vi "Client Loop Async.vi"(11 "VISA Client in":refnum<class "Serial Client.lvclass">) -> ()   [LabVIEW 2020, in "Stream-Serial.lvlib" / "Serial Client.lvclass"]
uses:
  Serial Client.lvclass
  C:/Program Files (x86)/National Instruments/LabVIEW 2020/vi.lib/IlluminatedG/lv-stream/Connection/Connection.lvclass
  C:/Program Files (x86)/National Instruments/LabVIEW 2020/vi.lib/IlluminatedG/lv-stream/Endpoint/Endpoint.lvclass
  Port Config.ctl
  Stop Bits.ctl
  Flow Control.ctl
  Parity.ctl
  <vilib>/IlluminatedG/lv-stream/Connection/State.ctl
  <vilib>/IlluminatedG/lv-stream/Connection State.ctl
  Client Command.ctl
  <vilib>/IlluminatedG/lv-stream/Endpoint/Endpoint.lvclass
  <vilib>/IlluminatedG/lv-stream/Connection/Connection.lvclass
  <vilib>/IlluminatedG/lv-stream/Stream.lvlib
  Stream-Serial.lvlib
panel:
  out "State":T1
  out "Port Config":T2={"Baud (115200)"=115200, "Data Bits (8)"=8, "Stop Bits (1)"=10, "Flow Control"=0, "Use LineTerm?"=FALSE, "LineTerm (\\n)"="\n", "Timeout ms (10000)"=10000, "Parity (None)"=enum."None"} {"Flow Control" items=["None", "XON/XOFF", "RTS/CTS", "XON/XOFF & RTS/CTS", "DTR/DSR", "XON/XOFF & DTR/DSR"]; "Stop Bits (1)" items=["1.0"=10, "1.5"=15, "2.0"=20]}
  out "Resource":string
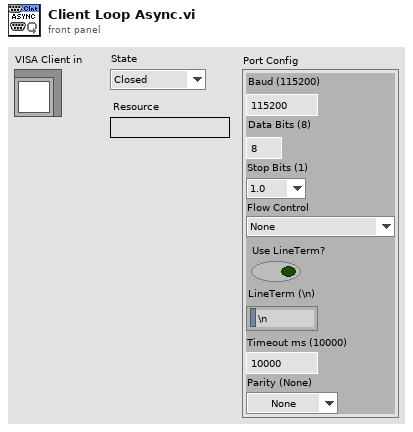
[diagram p1: front panel]
types:
  T1 = typedef "Stream.lvlib/Connection.lvclass/State.ctl" = enum16{"Closed", "Idle", "Connecting", "Connected", "Shutdown"}
  T2 = typedef "Stream-Serial.lvlib/Serial Client.lvclass/Port Config.ctl" = cluster{"Baud (115200)":u32, "Data Bits (8)":u8, "Stop Bits (1)":T3, "Flow Control":T4, "Use LineTerm?":bool, "LineTerm (\\n)":string, "Timeout ms (10000)":i32, "Parity (None)":T5}
  T3 = typedef "Stream-Serial.lvlib/Serial Client.lvclass/Stop Bits.ctl" = u16
  T4 = typedef "Stream-Serial.lvlib/Serial Client.lvclass/Flow Control.ctl" = u16
  T5 = typedef "Stream-Serial.lvlib/Serial Client.lvclass/Parity.ctl" = enum16{"None", "Odd", "Even", "Mark", "Space"}
  T6 = typedef "Stream.lvlib/Connection State.ctl" = enum16{"Connected", "Disconnected"}
  T7 = typedef "Stream-Serial.lvlib/Client Command.ctl" = enum16{"Connect", "Close", "Shutdown", "Reconnect"}
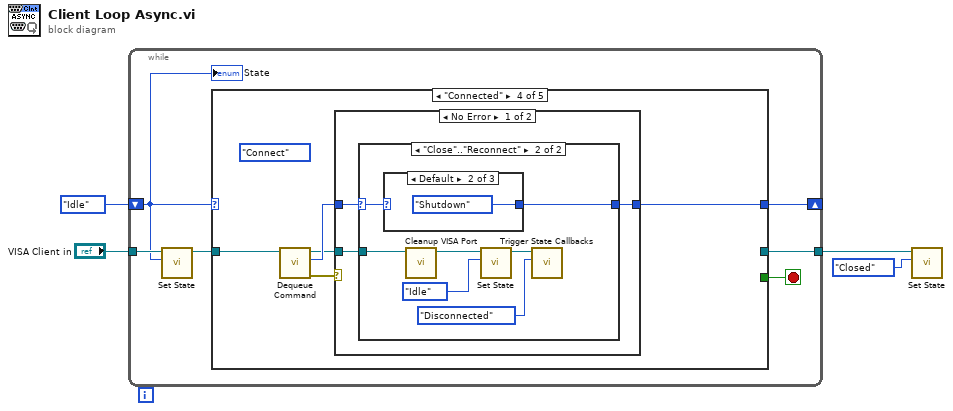
[diagram p0: block diagram]
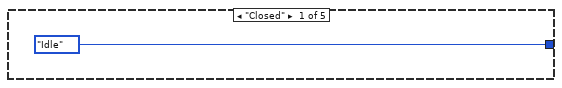
[diagram p2: hidden frame]
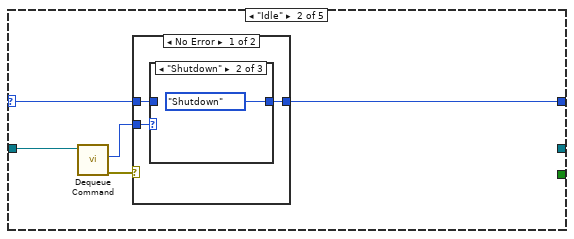
[diagram p3: hidden frame]
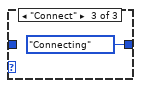
[diagram p5: hidden frame]
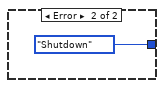
[diagram p6: hidden frame]
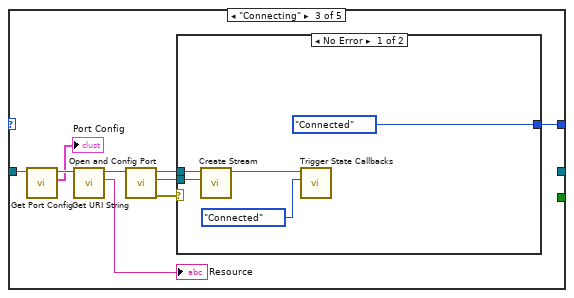
[diagram p7: hidden frame]
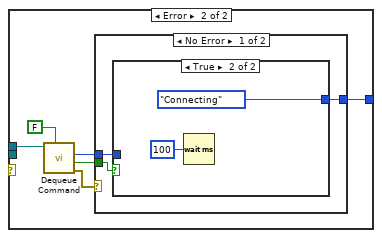
[diagram p8: hidden frame]
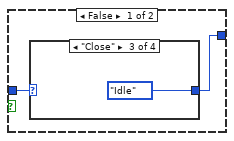
[diagram p9: hidden frame]
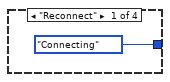
[diagram p10: hidden frame]
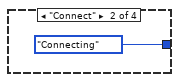
[diagram p11: hidden frame]
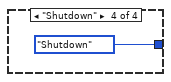
[diagram p12: hidden frame]
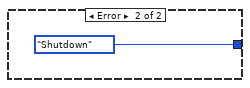
[diagram p13: hidden frame]
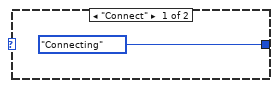
[diagram p14: hidden frame]
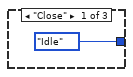
[diagram p15: hidden frame]
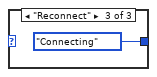
[diagram p16: hidden frame]
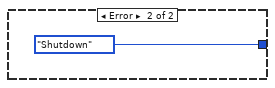
[diagram p17: hidden frame]
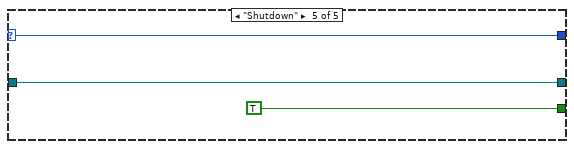
[diagram p18: hidden frame]
diagram:
  n1 = while {
    tunnel: "VISA Client in" -> [w7]
    shift-right: [w10] -> _
    shift-left: State."Idle" ("State") -> [w5]
    tunnel: [w9] -> w2
    stop <- w8 stop-if-true
    n2 = call <vilib>:"Set State.vi"("State"=w5, "Connection in"=w7) -> ("Connection out"=w6:refnum<class "Serial Client.lvclass">)  [unwired: 8 in, 1 out]
    n3 = case shown="\"Connected\"" w5 {
      selector: w5 -> [_ w14 _ _ w77]
      tunnel: w6 -> [_ w16 w26 w60 w78]
      tunnel: [State."Idle" ("State") w13 w27 w56 w77] -> w10
      tunnel: [_ _ _ _ w78] -> w9
      tunnel: [_ _ _ _ TRUE] -> w8
      frame "Closed" {
      }
      frame "Idle" {
        n4 = call "Dequeue Command.vi"("VISA Client in"=w16) -> ("error out"=w12:errorcluster, "Command"=w15:T7)  [unwired: 7 in, 2 out]
        n5 = case shown="No Error" w12 {
          tunnel: w15 -> [w19 _]
          tunnel: w14 -> [w18 _]
          tunnel: [w17 State."Shutdown" ("State")] -> w13
          frame No Error {
            n6 = case shown="\"Shutdown\"" w19 {
              tunnel: w18 -> [w20 _ _]
              tunnel: [w20 State."Shutdown" ("State") State."Connecting" ("State")] -> w17
              frame Default {
              }
              frame "Shutdown" {
              }
              frame "Connect" {
              }
            }
          }
          frame Error {
          }
        }
      }
      frame "Connecting" {
        n7 = call "Get Port Config.vi"("Serial Client in"=w26) -> ("Port Config"=→"Port Config":T2, "Serial Client out"=w25:refnum<class "Serial Client.lvclass">)  [unwired: 8 in, 1 out]
        n8 = call <vilib>:"Get URI String.vi"("Endpoint in"=w25) -> ("URI String"=→"Resource":string, "Endpoint out"=w31:refnum<class "Serial Client.lvclass">)  [unwired: 8 in, 1 out]
        n9 = call "Open and Config Port.vi"("Serial Client in"=w31) -> ("error out"=w30:errorcluster, "VISA resource name out"=w29:refnum<visa-resource-name>, "Serial Client"=w28:refnum<class "Serial Client.lvclass">)  [unwired: 8 in]
        n10 = case shown="No Error" w30 {
          tunnel: w29 -> [w35 _]
          tunnel: w28 -> [w36 w43]
          tunnel: [State."Connected" ("State") w38] -> w27
          frame No Error {
            n11 = call "Create Stream.vi"("VISA resource name"=w35, "Serial Client in"=w36) -> ("Serial Client out"=w34:refnum<class "Serial Client.lvclass">)  [unwired: 8 in, 1 out]
            n12 = call <vilib>:"Trigger State Callbacks.vi"("State"=Connection_State."Connected", "Connection in"=w34) -> ()  [unwired: 8 in, 2 out]
          }
          frame Error {
            n13 = call "Dequeue Command.vi"("Wait? (T)"=FALSE, "VISA Client in"=w43) -> ("error out"=w41:errorcluster, "Timed Out"=w40:bool, "Command"=w39:T7)  [unwired: 6 in, 1 out]
            n14 = case shown="No Error" w41 {
              tunnel: w40 -> [w46 _]
              tunnel: w39 -> [w45 _]
              tunnel: [w44 State."Shutdown" ("State")] -> w38
              frame No Error {
                n15 = case shown="True" w46 {
                  tunnel: w45 -> [w48 _]
                  tunnel: [w47 State."Connecting" ("State")] -> w44
                  frame False {
                    n16 = case shown="\"Close\"" w48 {
                      tunnel: [State."Connecting" ("State") State."Connecting" ("State") State."Idle" ("State") State."Shutdown" ("State")] -> w47
                      frame "Reconnect" {
                      }
                      frame "Connect" {
                      }
                      frame "Close" {
                      }
                      frame "Shutdown" {
                      }
                    }
                  }
                  frame True {
                    n17 = Wait (ms)(milliseconds to wait=u32 100) -> ()  [unwired: 1 out]
                  }
                }
              }
              frame Error {
              }
            }
          }
        }
      }
      frame "Connected" {
        (unwired) Client_Command."Connect" ("Command")
        n18 = call "Dequeue Command.vi"("VISA Client in"=w60) -> ("error out"=w59:errorcluster, "Command"=w58:T7, "VISA Client out"=w57:refnum<class "Serial Client.lvclass">)  [unwired: 7 in, 1 out]
        n19 = case shown="No Error" w59 {
          tunnel: w58 -> [w63 _]
          tunnel: w57 -> [w62 _]
          tunnel: [w61 State."Shutdown" ("State")] -> w56
          frame No Error {
            n20 = case shown="\"Close\"..\"Reconnect\"" w63 {
              selector: w63 -> [_ w69]
              tunnel: w62 -> [_ w71]
              tunnel: [State."Connecting" ("State") w68] -> w61
              frame "Connect" {
              }
              frame "Close".."Reconnect" {
                n21 = case shown="Default" w69 {
                  tunnel: [State."Idle" ("State") State."Shutdown" ("State") State."Connecting" ("State")] -> w68
                  frame "Close" {
                  }
                  frame Default {
                  }
                  frame "Reconnect" {
                  }
                }
                n22 = call "Cleanup VISA Port.vi"("Serial Client in"=w71) -> ("Serial Client out"=w67:refnum<class "Serial Client.lvclass">)  [unwired: 9 in, 1 out]
                n23 = call <vilib>:"Set State.vi"("State"=State."Idle", "Connection in"=w67) -> ("Connection out"=w65:refnum<class "Serial Client.lvclass">)  [unwired: 8 in, 1 out]
                n24 = call <vilib>:"Trigger State Callbacks.vi"("State"=Connection_State."Disconnected", "Connection in"=w65) -> ()  [unwired: 8 in, 2 out]
              }
            }
          }
          frame Error {
          }
        }
      }
      frame "Shutdown" {
      }
    }
    "State" <- w5
  }
  n25 = call <vilib>:"Set State.vi"("State"=State."Closed", "Connection in"=w2) -> ()  [unwired: 8 in, 2 out]
